vi "Write Function Name.vi"(8 "error in (no error)":errorcluster, 10 "Function Name":string, 11 "Select a function Msg in":refnum<class "Select a function Msg.lvclass">) -> (0 "error out":errorcluster, 3 "Select a function Msg out":refnum<class "Select a function Msg.lvclass">)   [LabVIEW 2016, in "Controller UI.lvlib" / "Select a function Msg.lvclass"]
uses:
  <userlib>/Common Components/Controller UI Messages/Select a function Msg/Select a function Msg.lvclass
  <userlib>/Common Components/Controller UI Messages/Select a function Msg/Select a function Msg.lvclass/Select a function Msg.ctl
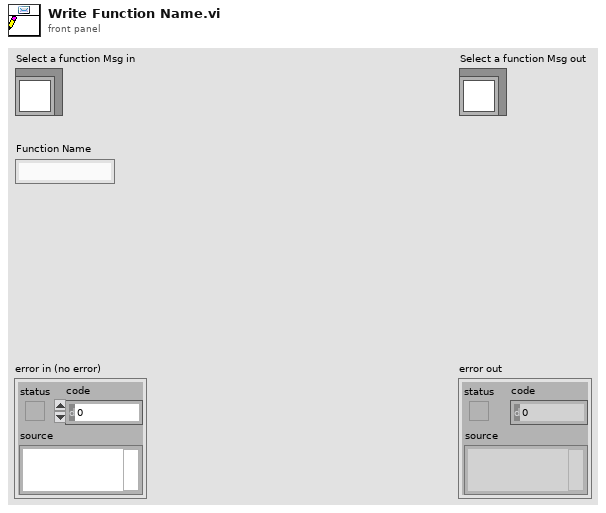
[diagram p1: front panel]
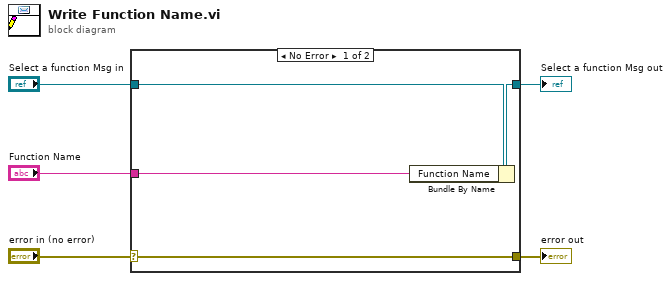
[diagram p0: block diagram]
diagram:
  n1 = case shown="No Error" "error in (no error)" {
    selector: "error in (no error)" -> [w9 w10]
    tunnel: [w9 w10] -> w4
    tunnel: [w7 w11] -> w2
    tunnel: "Select a function Msg in" -> [w8 w11]
    tunnel: "Function Name" -> [w6 _]
    frame No Error {
      n2 = Bundle By Name(cluster=w8, "Function Name"=w6) -> (w7:refnum<class "Select a function Msg.lvclass">)
    }
    frame Error {
    }
  }
  "error out" <- w4
  "Select a function Msg out" <- w2
